vi "File_Write_v2.vi"(0 "Thermocouple Data":dynamicdata(waveform), 1 "Pressure Data":T7, 2 "Use Older File Write?":bool, 3 "Flow Rate Data":cluster{dbl, dbl, dbl, dbl, dbl}, 4 "Raman Data Array":cluster{i32[], i32[]}[](array[cluster]), 5 "Loop Iteration Boolean":bool, 6 "Slave Data Cluster":T5={"Current DoE"=[], "SSI 1 Flow Rate"=0.0, "SSI 2 Flow Rate"=0.0, "FLOM 1 Flow Rate"=0.0, "FLOM 2 Flow Rate"=0.0, "Pumps Running?"=FALSE, "Boolean 2"=FALSE, "Boolean 3"=FALSE, "Boolean 4"=FALSE, "At Equilibrium?"=FALSE, "Script Running?"=FALSE, "Current Script Iteration"=0.0, "Total Script Iterations"=0.0, "FLOM Pumps VISA"="COM2", "SSI 1 Pump VISA"="COM76", "SSI 2 Pump VISA"="COM74", "Huber Unistat VISA"="COM1", "SSI 3 Pump VISA"="COM76", "SSI 4 Pump VISA"="COM76", "SSI 4 Flow Rate"=0.0, "SSI 3 Flow Rate"=0.0, "Flow Meter 1 Rate "=0.0, "Flow Meter 2 Rate"=0.0, "Flow Meter 3 Rate"=0.0, "Flow Meter 4 Rate"=0.0, "SSI 1 Flow Setpoint"=0.0, "SSI 2 Flow Setpoint"=0.0, "SSI 3 Flow Setpoint"=0.0, "SSI 4 Flow Setpoint"=0.0, "Temperature Setpoint"=0.0, "Flow meter 3 COM"=17, "Flow meter 5 COM"=18, "Flow meter 4 COM"=19, "Flow meter 2 COM"=16, "Flow meter 1 COM"=15, "Unit"=enum."PSI", "Pressure COM"="COM6", "Julabo Setpoint"=0.0, "Julabo Control"=enum."Internal", "Overtemp"=50.0, "Subtemp"=-20.0, "HeatMax"=50, "CoolMax"=-100, "InternMax"=50.0, "InternMin"=0.0, "Upper Bandlimit"=100.0, "Lower Bandlimit"=0.0, "Julabo CF41 VISA"="COM3", "Xp (0.6K) Int"=0.6, "Tn (3s) Int"=3, "Tv (0s) Int"=0, "Dynamic (0: aperiodic) Int"=enum."aperiodic", "Xp (0.6K) Ext"=0.6, "Tn (3s) Ext"=3, "Tv (0s) Ext"=0, "XpU (0.6K) Ext"=0.6, "Julabo Serial Configuration"={"Baud Rate"=4800, "Parity"=2, "Data Bits"=7, "Stop Bits"=10, "Flow Control"=2}} {"Julabo Serial Configuration"."Flow Control" items=["None", "XON/XOFF", "RTS/CTS", "XON/XOFF & RTS/CTS", "DTR/DSR", "XON/XOFF & DTR/DSR"]; "Julabo Serial Configuration"."Stop Bits" items=["1.0"=10, "1.5"=15, "2.0"=20]; "Julabo Serial Configuration"."Data Bits" items=["7"=7, "8"=8]; "Julabo Serial Configuration"."Parity" items=["None", "Odd", "Even", "Mark", "Space"]; "Julabo Serial Configuration"."Baud Rate" items=["300"=300, "600"=600, "1200"=1200, "2400"=2400, "4800"=4800, "9600"=9600, "19200"=19200]; "XpU (0.6K) Ext" min=0.1 max=99.9; "Tv (0s) Ext" max=999; "Tn (3s) Ext" min=3 max=9999; "Xp (0.6K) Ext" min=0.1 max=99.9; "Tv (0s) Int" max=999; "Tn (3s) Int" min=3 max=9999; "Xp (0.6K) Int" min=0.1 max=99.9; "Lower Bandlimit" min=0.0 max=200.0; "Upper Bandlimit" min=0.0 max=200.0; "InternMin" format="%.2f"; "InternMax" format="%.2f"; "CoolMax" min=-100 max=0; "HeatMax" max=100; "Subtemp" format="%.2f"; "Overtemp" format="%.2f"; "Julabo Setpoint" format="%.2f"; "Current DoE" format="%0.3f"}, 8 "File Path Cluster":T4, 10 "Julabo Outputs":T1, 12 "Numeric":i32, 13 "Array":i32[](array[numeric]), 14 "Thermocouple T-Plots":T3(graph), 16 "dT/dt":cluster{"dx/dt":dbl, "dx/dt":dbl, "dx/dt":dbl}(graph), 18 "dF/dt":T2(graph)) -> (15 "Data_Reactant 1 path":path caption="selected path", 17 "Data_Reactant 2 path":path caption="selected path", 20 "Filepath Cluster Out":T4, 24 "Data_noRaman path":path caption="selected path", 25 "Data_Product path":path caption="selected path", 27 "Data_Reactant 3 path":path caption="selected path")   [LabVIEW 2015]
uses:
  --Controls and TypeDefs--/DoE_Control_Cluster.ctl
  <instrlib>/JULABO DeviceDriver/Examples/Julabo Serial Control.ctl
  <vilib>/Utility/file.llb/Write To Spreadsheet File (string).vi
panel:
  in  "Write Raman-Appended Files?":bool
  in  "data File Header":string[][](table)=[["Time"], ["TC1"], ["TC2"], ["TC3"], ["TC1 SG Filter"], ["TC2 SG Filter"], ["TC3 SG Filter"], ["TC1 dT/dt"], ["TC2 dT/dt"], ["TC3 dT/dt"], ["P1"], ["P2"], ["P3"], ["P4"], ["Fset1"], ["Fset2"], ["Fset3"], ["Fset4"], ["F1"], ["F2"], ["F3"], ["F4"], ["F5"], ["F1 dF/dt"], ["F2 dF/dt"], ["F3 dF/dt"], ["F4 dF/dt"], ["F5 dF/dt"]]
  # "Julabo"
  # "Limits"
  # "PID Control Parameters"
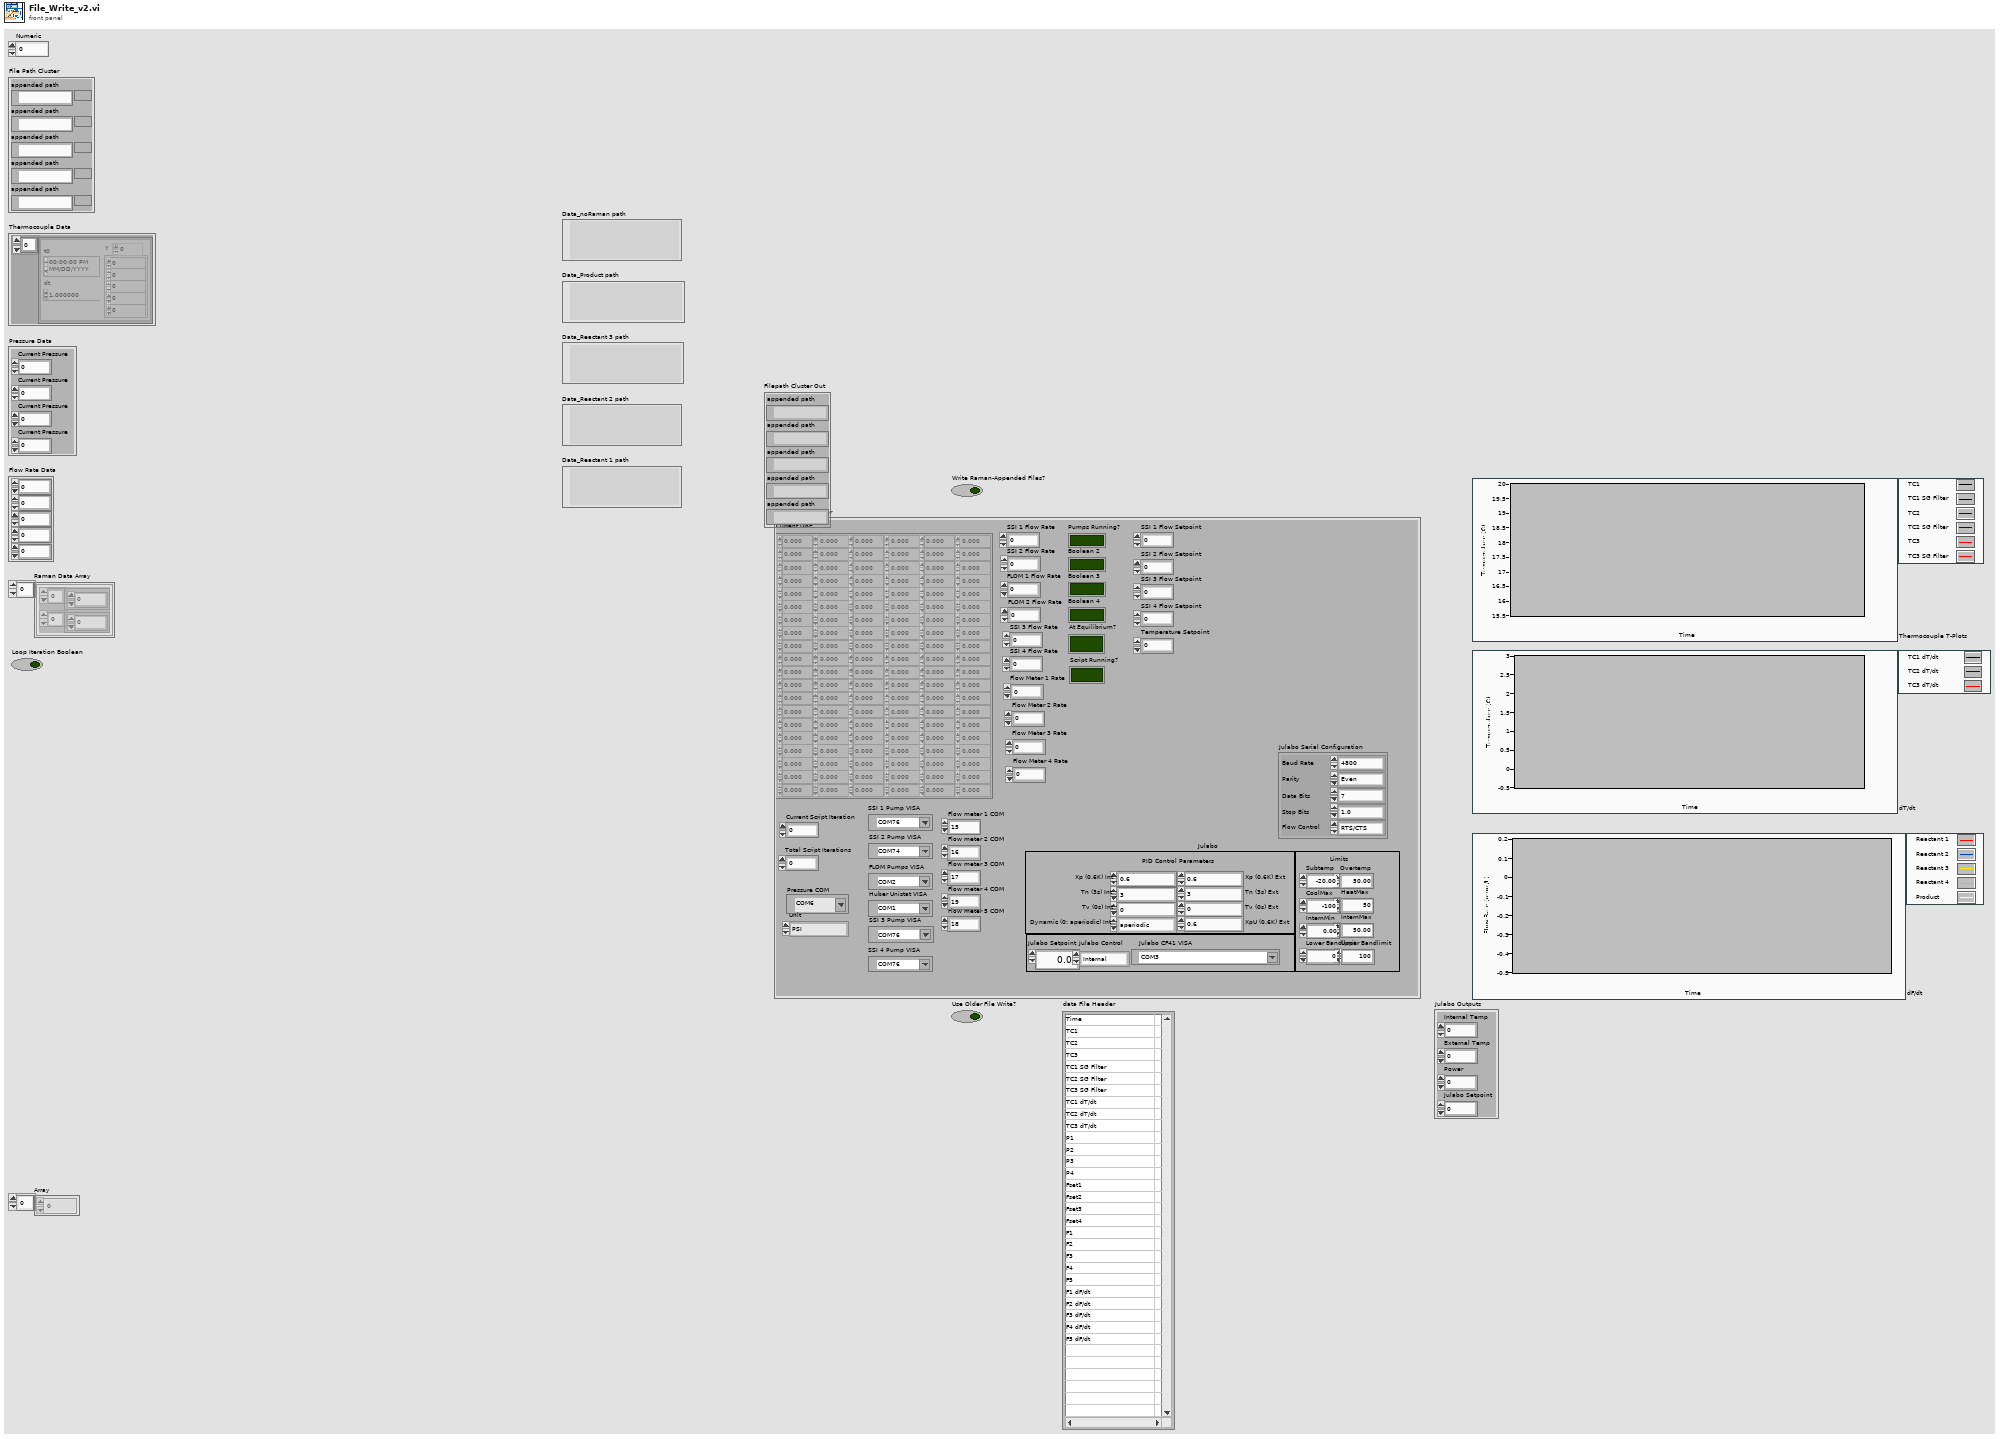
[diagram p1: front panel]
types:
  T1 = cluster{"Internal Temp":dbl, "External Temp":dbl, "Power":i8, "Julabo Setpoint":dbl}
  T2 = cluster{"MeasureResult Scaled":dbl, "MeasureResult Scaled":dbl, "MeasureResult Scaled":dbl, "MeasureResult Scaled":dbl, "MeasureResult Scaled":dbl}
  T3 = cluster{dbl, "Filtered x":dbl, dbl, "Filtered x":dbl, dbl, "Filtered x":dbl}
  T4 = cluster{"appended path":path, "appended path":path, "appended path":path, "appended path":path, "appended path":path}
  T5 = typedef "DoE_Control_Cluster.ctl" = cluster{"Current DoE":dbl[][], "SSI 1 Flow Rate":dbl, "SSI 2 Flow Rate":dbl, "FLOM 1 Flow Rate":dbl, "FLOM 2 Flow Rate":dbl, "Pumps Running?":bool, "Boolean 2":bool, "Boolean 3":bool, "Boolean 4":bool, "At Equilibrium?":bool, "Script Running?":bool, "Current Script Iteration":dbl, "Total Script Iterations":dbl, "FLOM Pumps VISA":refnum<visa-resource-name>, "SSI 1 Pump VISA":refnum<visa-resource-name>, "SSI 2 Pump VISA":refnum<visa-resource-name>, "Huber Unistat VISA":refnum<visa-resource-name>, "SSI 3 Pump VISA":refnum<visa-resource-name>, "SSI 4 Pump VISA":refnum<visa-resource-name>, "SSI 4 Flow Rate":dbl, "SSI 3 Flow Rate":dbl, "Flow Meter 1 Rate ":dbl, "Flow Meter 2 Rate":dbl, "Flow Meter 3 Rate":dbl, "Flow Meter 4 Rate":dbl, "SSI 1 Flow Setpoint":dbl, "SSI 2 Flow Setpoint":dbl, "SSI 3 Flow Setpoint":dbl, "SSI 4 Flow Setpoint":dbl, "Temperature Setpoint":dbl, "Flow meter 3 COM":u16, "Flow meter 5 COM":u16, "Flow meter 4 COM":u16, "Flow meter 2 COM":u16, "Flow meter 1 COM":u16, "Unit":enum16{"PSI", "Bar", "cm H2O", "ft H2O", "hectoPascal", "in Hg", "in H2O", "kiloPascal", "milliBar", "mmHg", "MegaPascal", "Numeric Pressure"}, "Pressure COM":refnum<visa-resource-name>, "Julabo Setpoint":dbl, "Julabo Control":enum16{"Internal", "External"}, "Overtemp":dbl, "Subtemp":dbl, "HeatMax":u8, "CoolMax":i8, "InternMax":dbl, "InternMin":dbl, "Upper Bandlimit":dbl, "Lower Bandlimit":dbl, "Julabo CF41 VISA":refnum<visa-resource-name>, "Xp (0.6K) Int":dbl, "Tn (3s) Int":u16, "Tv (0s) Int":u16, "Dynamic (0: aperiodic) Int":enum16{"aperiodic", "standard"}, "Xp (0.6K) Ext":dbl, "Tn (3s) Ext":u16, "Tv (0s) Ext":u16, "XpU (0.6K) Ext":dbl, "Julabo Serial Configuration":T6}
  T6 = typedef "Julabo Serial Control.ctl" = cluster{"Baud Rate":u32, "Parity":u16, "Data Bits":u16, "Stop Bits":u16, "Flow Control":u16}
  T7 = cluster{"Current Pressure":dbl, "Current Pressure":dbl, "Current Pressure":dbl, "Current Pressure":dbl}
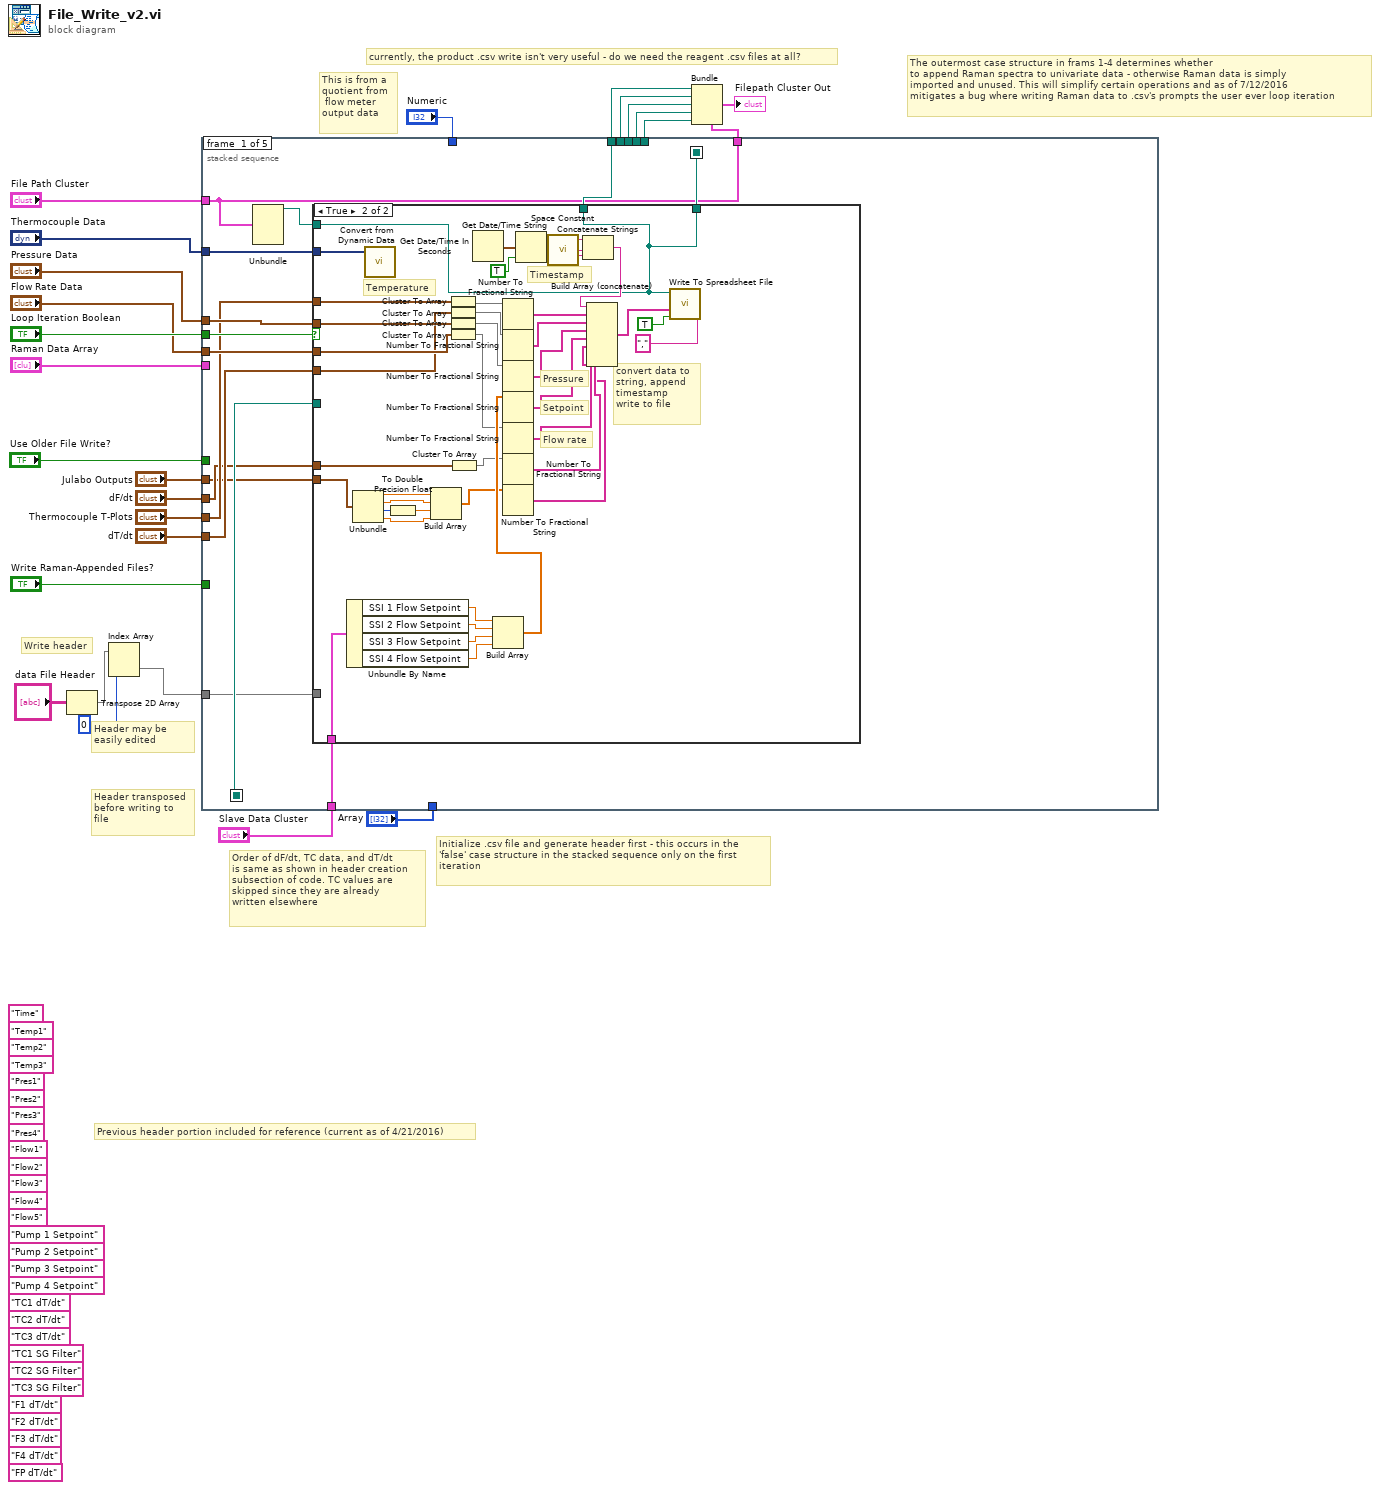
[diagram p0: block diagram]
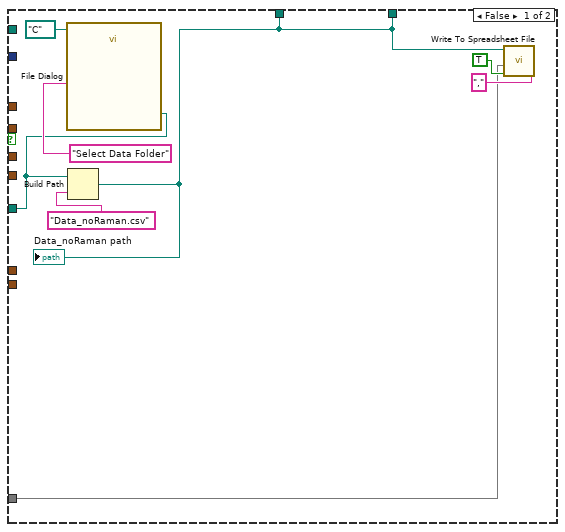
[diagram p2: hidden frame]
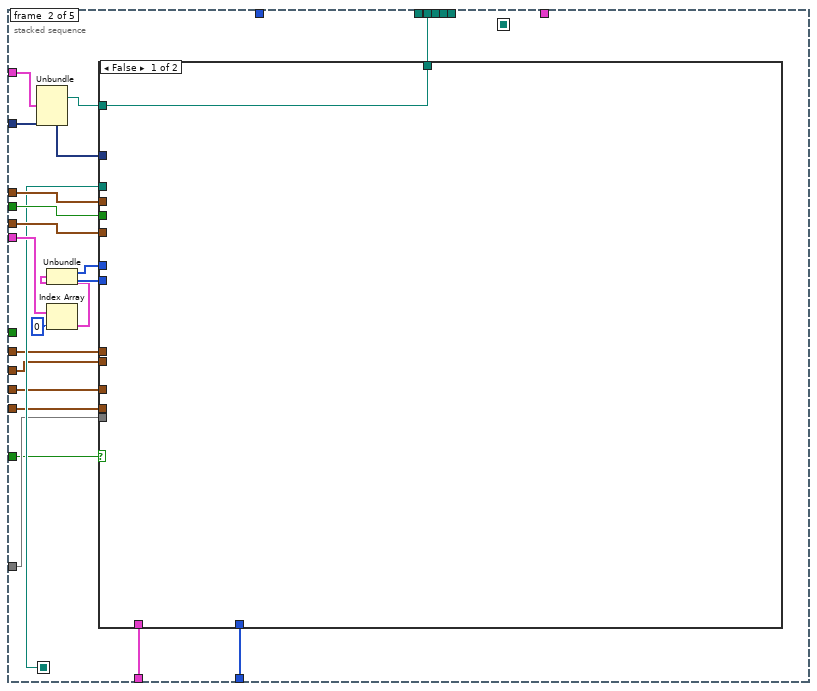
[diagram p3: hidden frame]
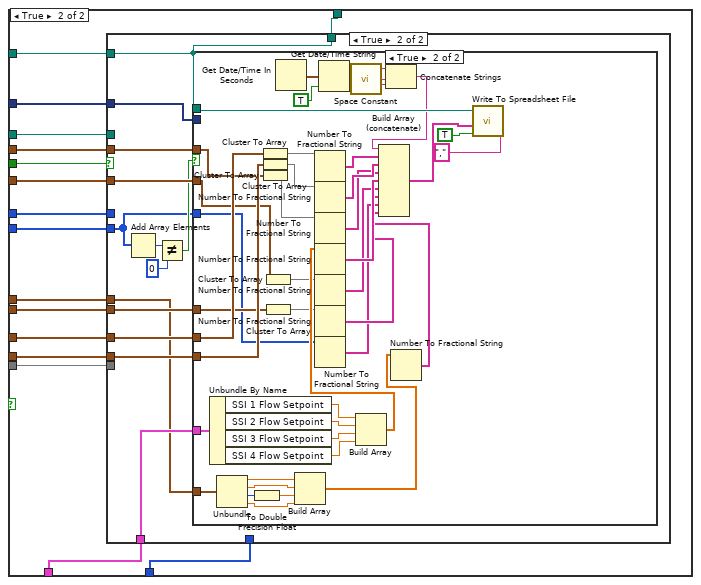
[diagram p4: hidden frame]
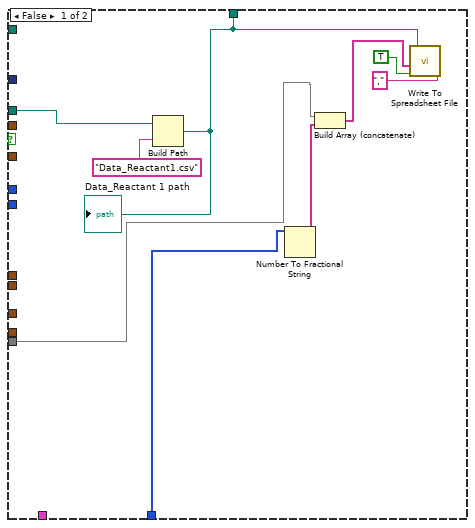
[diagram p5: hidden frame]
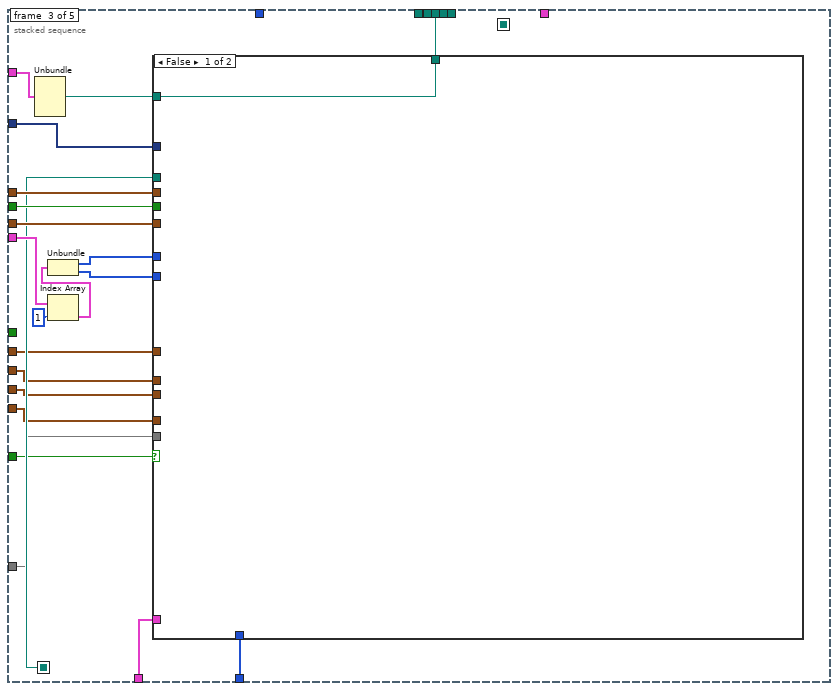
[diagram p7: hidden frame]
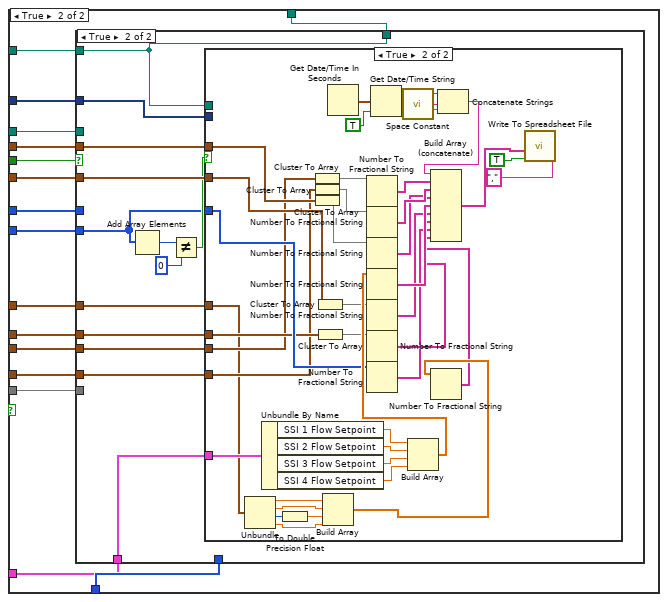
[diagram p8: hidden frame]
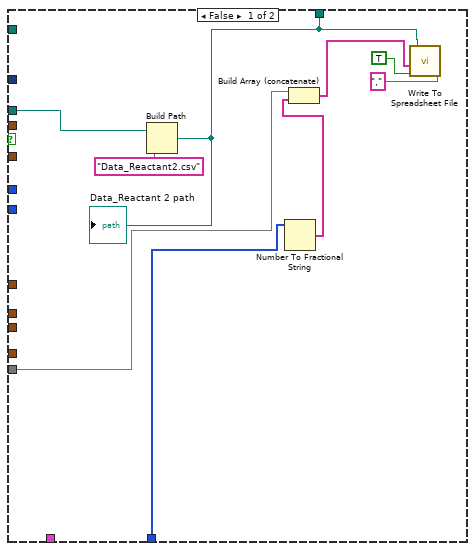
[diagram p9: hidden frame]
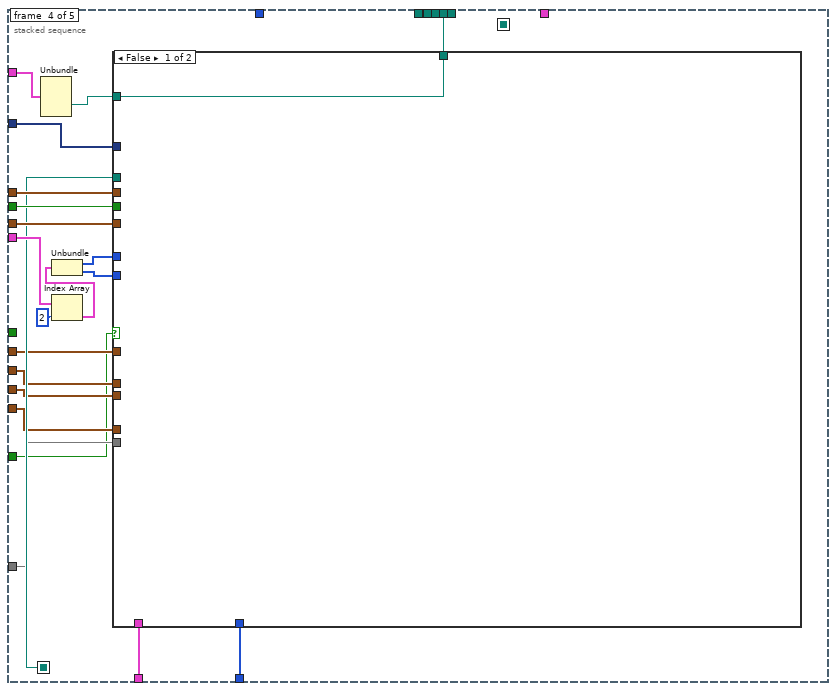
[diagram p11: hidden frame]
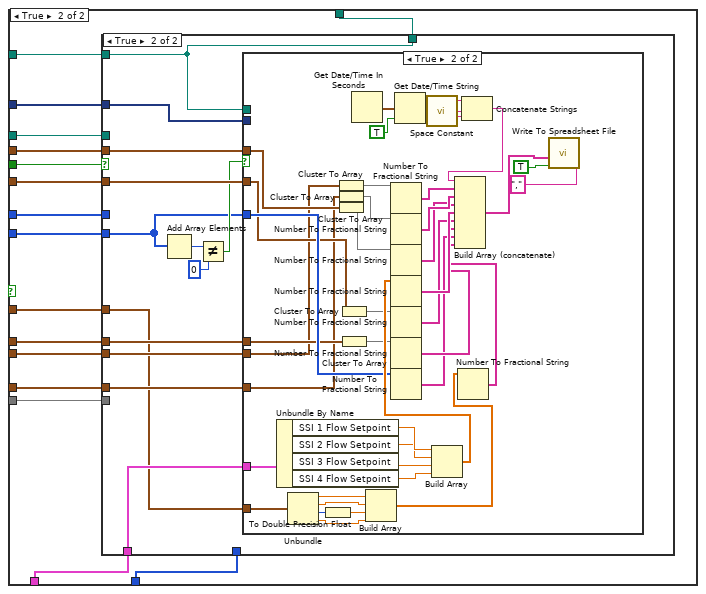
[diagram p12: hidden frame]
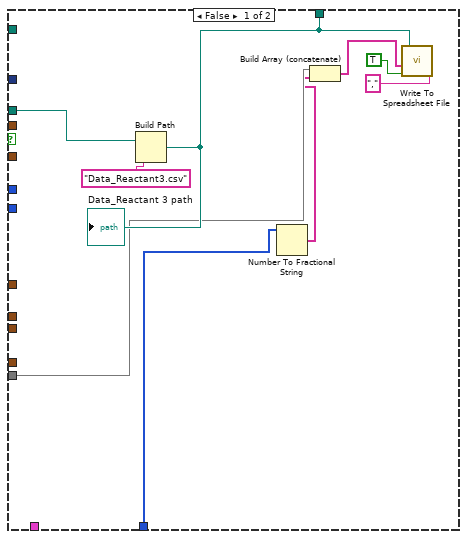
[diagram p13: hidden frame]
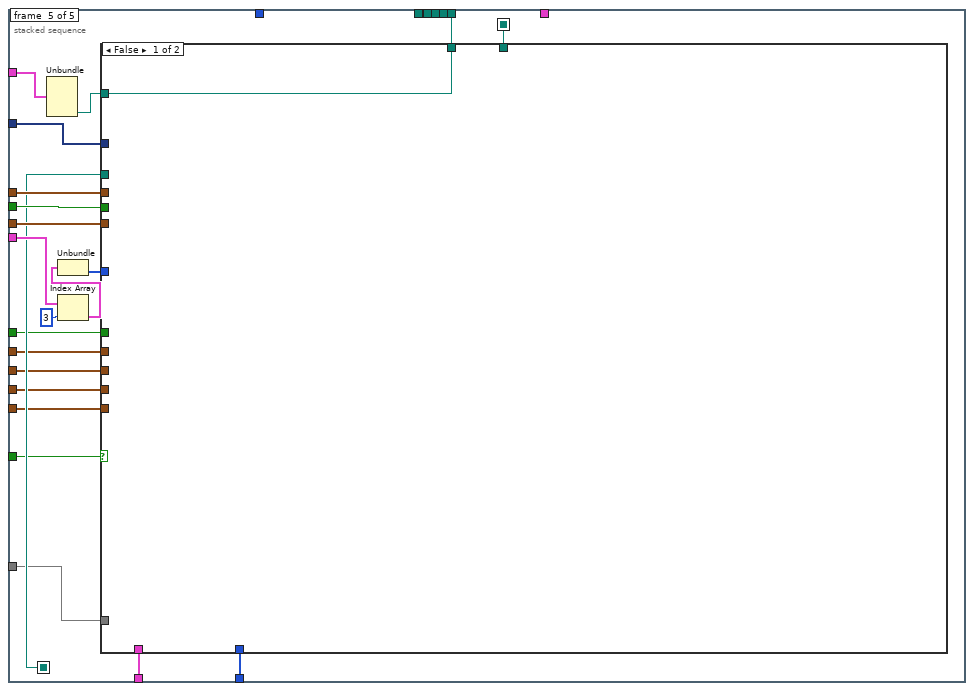
[diagram p15: hidden frame]
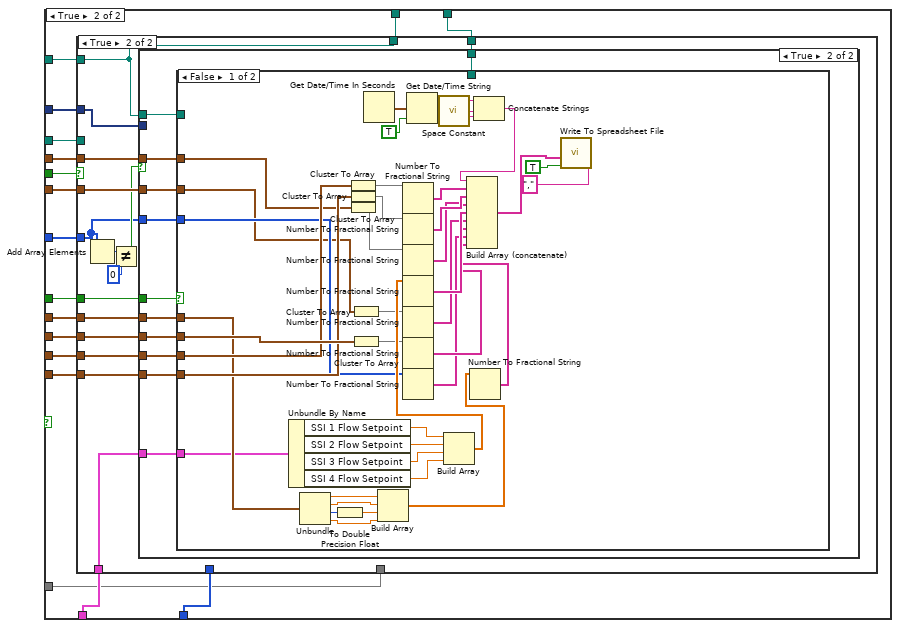
[diagram p16: hidden frame]
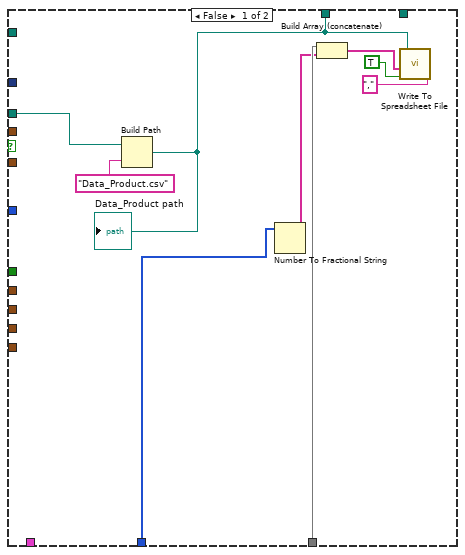
[diagram p17: hidden frame]
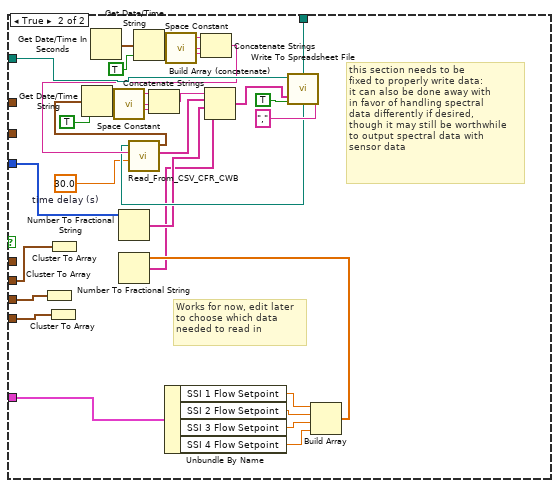
[diagram p19: hidden frame]
diagram:
  (unwired) "FP dT/dt"
  (unwired) "F4 dT/dt"
  (unwired) "F3 dT/dt"
  (unwired) "F2 dT/dt"
  (unwired) "F1 dT/dt"
  (unwired) "TC2 SG Filter"
  (unwired) "TC3 SG Filter"
  (unwired) "TC1 SG Filter"
  (unwired) "TC3 dT/dt"
  (unwired) "TC2 dT/dt"
  (unwired) "TC1 dT/dt"
  (unwired) "Pump 4 Setpoint"
  (unwired) "Pump 3 Setpoint"
  (unwired) "Pump 2 Setpoint"
  (unwired) "Pump 1 Setpoint"
  (unwired) "Flow5" ("delimiter (\\t)")
  (unwired) "Flow4" ("delimiter (\\t)")
  (unwired) "Flow3" ("delimiter (\\t)")
  (unwired) "Flow2" ("delimiter (\\t)")
  (unwired) "Flow1" ("delimiter (\\t)")
  (unwired) "Pres4" ("delimiter (\\t)")
  (unwired) "Pres3" ("delimiter (\\t)")
  (unwired) "Pres2" ("delimiter (\\t)")
  (unwired) "Pres1" ("delimiter (\\t)")
  (unwired) "Temp3" ("delimiter (\\t)")
  (unwired) "Temp2" ("delimiter (\\t)")
  (unwired) "Temp1" ("delimiter (\\t)")
  (unwired) "Time" ("delimiter (\\t)")
  # "The outermost case structure in frams 1-4 determines whether\nto append Raman spectra to univariate data - otherwise Raman data is simply\nimported and unused. This will simplify certain operations and as of 7/12/2016 \nmitigates a bug where writing Raman data to .csv's prompts the user ever loop iteration"
  # "currently, the product .csv write isn't very useful - do we need the reagent .csv files at all?"
  # "Write header"
  # "Previous header portion included for reference (current as of 4/21/2016)"
  # "Header transposed\nbefore writing to \nfile"
  # "Header may be \neasily edited"
  # "Order of dF/dt, TC data, and dT/dt \nis same as shown in header creation \nsubsection of code. TC values are\nskipped since they are already\nwritten elsewhere"
  # "Initialize .csv file and generate header first - this occurs in the 'false' case structure in the stacked sequence only on the first iteration"
  # "This is from a \nquotient from\n flow meter\noutput data"
  n1 = Transpose 2D Array(2D array="data File Header") -> (transposed array=w6:string[][])
  n2 = Index Array(array=w6, index (row)=0) -> (element=w5:string[])  [unwired: 1 in]
  n3 = stacked-sequence {
    seq-local: [w36 _ _ _ _] -> [_ w99 w201 w302 w405]
    seq-local: [w35 _ _ _ _] -> [_ _ _ _ w403]
    tunnel: "Thermocouple Data" -> [w37 w111 w213 w314 w416]
    tunnel: "Pressure Data" -> [w41 w110 w212 w313 w415]
    tunnel: "Flow Rate Data" -> [w40 w109 w211 w312 w414]
    tunnel: "Loop Iteration Boolean" -> [w39 w108 w210 w311 w413]
    tunnel: [w33 _ _ _ _] -> w15
    tunnel: "File Path Cluster" -> [w32 w101 w203 w304 w407]
    tunnel: "Raman Data Array" -> [_ w105 w207 w308 w411]
    tunnel: [_ w102 _ _ _] -> w14
    tunnel: [_ _ w204 _ _] -> w13
    tunnel: [_ _ _ w305 _] -> w11
    tunnel: [_ _ _ _ w408] -> w12
    tunnel: "Array" -> [_ w98 w200 w301 w404]
    tunnel: "Numeric" -> [_ _ _ _ _]
    tunnel: "Slave Data Cluster" -> [w34 w97 w199 w300 w402]
    tunnel: [w32 _ _ _ _] -> w17
    tunnel: "dT/dt" -> [w29 w94 w196 w297 w401]
    tunnel: "Thermocouple T-Plots" -> [w30 w95 w195 w296 w400]
    tunnel: "dF/dt" -> [w28 w93 w197 w298 w399]
    tunnel: w5 -> [w31 w96 w198 w299 w398]
    tunnel: "Julabo Outputs" -> [w27 w92 w194 w295 w397]
    tunnel: "Use Older File Write?" -> [_ _ _ _ w396]
    tunnel: "Write Raman-Appended Files?" -> [_ w91 w193 w294 w395]
    frame #0 {
      n4 = Unbundle(w32) -> ("appended path"=w38:path)  [unwired: 4 out]
      n5 = case shown="True" w39 {
        tunnel: w37 -> [_ w79]
        tunnel: w41 -> [_ w78]
        tunnel: w40 -> [_ w77]
        tunnel: w38 -> [_ w76]
        tunnel: [w43 w76] -> w33
        tunnel: [w44 _] -> w36
        tunnel: [w43 w76] -> w35
        tunnel: w34 -> [_ w75]
        tunnel: w31 -> [w42 _]
        tunnel: w30 -> [_ w70]
        tunnel: w29 -> [_ w68]
        tunnel: w28 -> [_ w61]
        tunnel: w27 -> [_ w57]
        frame False {
          n6 = call "File Dialog"("start path"=path "C:/", "prompt"="Select Data Folder") -> ("selected path"=w44:path)  [unwired: 10 in, 3 out]
          n7 = Build Path(base path=w44, name or relative path="Data_noRaman.csv" ("default name")) -> (appended path=w43:path)
          "Data_noRaman path" <- w43
          n8 = call-poly <vilib>:"Write To Spreadsheet File.vi"("delimiter (\\t)"="," ("delimiter (\\t)"), "append to file? (new file:F)"=TRUE ("append to file?"), "1D data"=w42, "file path (dialog if empty)"=w43) -> ()  [unwired: 4 in, 1 out]
        }
        frame True {
          # "Timestamp"
          # "Setpoint"
          # "Temperature"
          # "Pressure"
          # "Flow rate"
          # "convert data to \nstring, append\ntimestamp\nwrite to file"
          n9 = Unbundle By Name(w75) -> ("SSI 1 Flow Setpoint"=w74:dbl, "SSI 2 Flow Setpoint"=w73:dbl, "SSI 3 Flow Setpoint"=w72:dbl, "SSI 4 Flow Setpoint"=w71:dbl)
          n10 = Unbundle(w57) -> ("Internal Temp"=w55:dbl, "External Temp"=w54:dbl, "Power"=w56:i8, "Julabo Setpoint"=w52:dbl)
          n11 = call "Convert from Dynamic Data"("Dynamic Data Type"=w79) -> ()  [unwired: 3 in, 1 out]
          n12 = To Double Precision Float(number=w56) -> (double precision float=w53:dbl)
          n13 = Build Array(w55, w54, w53, w52) -> (w51:dbl[])
          n14 = Cluster To Array(cluster=w70) -> (array=w69:dbl[])
          n15 = Cluster To Array(cluster=w68) -> (array=w67:dbl[])
          n16 = Cluster To Array(cluster=w78) -> (array=w88:dbl[])
          n17 = Cluster To Array(cluster=w77) -> (array=w64:dbl[])
          n18 = Cluster To Array(cluster=w61) -> (array=w60:dbl[])
          n19 = Get Date/Time In Seconds() -> (seconds since 1Jan1904=w82:timestamp)
          n20 = Build Array(w74, w73, w72, w71) -> (w65:dbl[])
          n21 = Number To Fractional String(number=w69) -> (F-format string=w89:string[])  [unwired: 3 in]
          n22 = Number To Fractional String(number=w67) -> (F-format string=w66:string[])  [unwired: 3 in]
          n23 = Number To Fractional String(number=w88) -> (F-format string=w63:string[])  [unwired: 3 in]
          n24 = Number To Fractional String(number=w65) -> (F-format string=w62:string[])  [unwired: 3 in]
          n25 = Number To Fractional String(number=w64) -> (F-format string=w59:string[])  [unwired: 3 in]
          n26 = Number To Fractional String(number=w60) -> (F-format string=w58:string[])  [unwired: 3 in]
          n27 = Number To Fractional String(number=w51) -> (F-format string=w50:string[])  [unwired: 3 in]
          n28 = Get Date/Time String(seconds (now)=w82, want seconds? (F)=TRUE) -> (date string=w84:string, time string=w85:string)  [unwired: 1 in]
          n29 = call <vilib>:"Space Constant.vi"() -> ("String"=w86:string)
          n30 = Concatenate Strings(w84, w86, w85) -> (w87:string)
          n31 = Build Array (concatenate)(w87, w89, w66, w63, w62, w59, w58, w50) -> (w90:string[])
          n32 = call-poly <vilib>:"Write To Spreadsheet File.vi"("delimiter (\\t)"="," ("delimiter (\\t)"), "append to file? (new file:F)"=TRUE ("append to file?"), "1D data"=w90, "file path (dialog if empty)"=w76) -> ()  [unwired: 4 in, 1 out]
        }
      }
    }
    frame #1 {
      n33 = Unbundle(w101) -> ("appended path"=w100:path)  [unwired: 4 out]
      n34 = Index Array(array=w105, index=0) -> (element=w104:cluster{i32[], i32[]})
      n35 = Unbundle(w104) -> (w106:i32[], w107:i32[])
      n36 = case shown="False" w91 {
        tunnel: w111 -> [_ w128]
        tunnel: w110 -> [_ w127]
        tunnel: w109 -> [_ w126]
        tunnel: w108 -> [_ w125]
        tunnel: w107 -> [_ w124]
        tunnel: w106 -> [_ w123]
        tunnel: [w112 w122] -> w102
        tunnel: w100 -> [w112 w121]
        tunnel: w99 -> [_ w120]
        tunnel: w98 -> [_ w119]
        tunnel: w97 -> [_ w118]
        tunnel: w96 -> [_ w117]
        tunnel: w95 -> [_ w116]
        tunnel: w94 -> [_ w115]
        tunnel: w93 -> [_ w114]
        tunnel: w92 -> [_ w113]
        frame False {
        }
        frame True {
          n37 = case shown="True" w125 {
            tunnel: w128 -> [_ w150]
            tunnel: w127 -> [_ w149]
            tunnel: w126 -> [_ w148]
            tunnel: w121 -> [_ w147]
            tunnel: [w137 w147] -> w122
            tunnel: w124 -> [_ w143]
            tunnel: w123 -> [_ _]
            tunnel: w120 -> [w136 _]
            tunnel: w119 -> [w132 _]
            tunnel: w118 -> [_ w142]
            tunnel: w117 -> [w131 _]
            tunnel: w116 -> [_ w141]
            tunnel: w115 -> [_ w140]
            tunnel: w114 -> [_ w139]
            tunnel: w113 -> [_ w138]
            frame False {
              n38 = Build Path(base path=w136, name or relative path="Data_Reactant1.csv" ("default name")) -> (appended path=w137:path)
              "Data_Reactant 1 path" <- w137
              n39 = Number To Fractional String(number=w132) -> (F-format string=w130:string[])  [unwired: 3 in]
              n40 = Build Array (concatenate)(w131, w130) -> (w129:string[])
              n41 = call-poly <vilib>:"Write To Spreadsheet File.vi"("delimiter (\\t)"="," ("delimiter (\\t)"), "append to file? (new file:F)"=TRUE ("append to file?"), "1D data"=w129, "file path (dialog if empty)"=w137) -> ()  [unwired: 4 in, 1 out]
            }
            frame True {
              n42 = Add Array Elements(numeric array=w143) -> (sum=w146:i32)
              n43 = Not Equal?(x=w146, y=0) -> (x != y?=w144:bool)
              n44 = case shown="True" w144 {
                tunnel: w150 -> [_ _]
                tunnel: w149 -> [_ w173]
                tunnel: w148 -> [_ w168]
                tunnel: w147 -> [_ w185]
                tunnel: w143 -> [_ w162]
                tunnel: w142 -> [_ w160]
                tunnel: w141 -> [_ w179]
                tunnel: w140 -> [_ w176]
                tunnel: w139 -> [_ w165]
                tunnel: w138 -> [_ w153]
                frame False {
                }
                frame True {
                  n45 = Unbundle By Name(w160) -> ("SSI 1 Flow Setpoint"=w184:dbl, "SSI 2 Flow Setpoint"=w183:dbl, "SSI 3 Flow Setpoint"=w182:dbl, "SSI 4 Flow Setpoint"=w181:dbl)
                  n46 = Unbundle(w153) -> ("Internal Temp"=w157:dbl, "External Temp"=w156:dbl, "Power"=w158:i8, "Julabo Setpoint"=w154:dbl)
                  n47 = To Double Precision Float(number=w158) -> (double precision float=w155:dbl)
                  n48 = Cluster To Array(cluster=w179) -> (array=w178:dbl[])
                  n49 = Cluster To Array(cluster=w176) -> (array=w175:dbl[])
                  n50 = Cluster To Array(cluster=w173) -> (array=w172:dbl[])
                  n51 = Cluster To Array(cluster=w168) -> (array=w167:dbl[])
                  n52 = Cluster To Array(cluster=w165) -> (array=w164:dbl[])
                  n53 = Get Date/Time In Seconds() -> (seconds since 1Jan1904=w188:timestamp)
                  n54 = Build Array(w157, w156, w155, w154) -> (w152:dbl[])
                  n55 = Number To Fractional String(number=w178) -> (F-format string=w177:string[])  [unwired: 3 in]
                  n56 = Number To Fractional String(number=w175) -> (F-format string=w174:string[])  [unwired: 3 in]
                  n57 = Number To Fractional String(number=w172) -> (F-format string=w171:string[])  [unwired: 3 in]
                  n58 = Number To Fractional String(number=w167) -> (F-format string=w166:string[])  [unwired: 3 in]
                  n59 = Number To Fractional String(number=w164) -> (F-format string=w163:string[])  [unwired: 3 in]
                  n60 = Number To Fractional String(number=w162) -> (F-format string=w161:string[])  [unwired: 3 in]
                  n61 = Get Date/Time String(seconds (now)=w188, want seconds? (F)=TRUE) -> (date string=w190:string, time string=w191:string)  [unwired: 1 in]
                  n62 = call <vilib>:"Space Constant.vi"() -> ("String"=w192:string)
                  n63 = Build Array(w184, w183, w182, w181) -> (w170:dbl[])
                  n64 = Number To Fractional String(number=w170) -> (F-format string=w169:string[])  [unwired: 3 in]
                  n65 = Concatenate Strings(w190, w192, w191) -> (w180:string)
                  n66 = Number To Fractional String(number=w152) -> (F-format string=w151:string[])  [unwired: 3 in]
                  n67 = Build Array (concatenate)(w180, w177, w174, w171, w169, w166, w163, w161, w151) -> (w159:string[])
                  n68 = call-poly <vilib>:"Write To Spreadsheet File.vi"("delimiter (\\t)"="," ("delimiter (\\t)"), "append to file? (new file:F)"=TRUE ("append to file?"), "1D data"=w159, "file path (dialog if empty)"=w185) -> ()  [unwired: 4 in, 1 out]
                }
              }
            }
          }
        }
      }
    }
    frame #2 {
      n69 = Unbundle(w203) -> ("appended path"=w202:path)  [unwired: 4 out]
      n70 = Index Array(array=w207, index=1) -> (element=w206:cluster{i32[], i32[]})
      n71 = Unbundle(w206) -> (w208:i32[], w209:i32[])
      n72 = case shown="False" w193 {
        tunnel: w213 -> [_ w230]
        tunnel: w212 -> [_ w229]
        tunnel: w211 -> [_ w228]
        tunnel: w210 -> [_ w227]
        tunnel: w209 -> [_ w226]
        tunnel: w208 -> [_ w225]
        tunnel: [w214 w224] -> w204
        tunnel: w202 -> [w214 w223]
        tunnel: w201 -> [_ w222]
        tunnel: w200 -> [_ w221]
        tunnel: w199 -> [_ w220]
        tunnel: w198 -> [_ w219]
        tunnel: w197 -> [_ w218]
        tunnel: w196 -> [_ w217]
        tunnel: w195 -> [_ w216]
        tunnel: w194 -> [_ w215]
        frame False {
        }
        frame True {
          n73 = case shown="True" w227 {
            tunnel: w230 -> [_ w252]
            tunnel: w229 -> [_ w251]
            tunnel: w228 -> [_ w250]
            tunnel: w223 -> [_ w249]
            tunnel: [w239 w249] -> w224
            tunnel: w226 -> [_ w245]
            tunnel: w225 -> [_ _]
            tunnel: w222 -> [w238 _]
            tunnel: w221 -> [w234 _]
            tunnel: w220 -> [_ w244]
            tunnel: w219 -> [w233 _]
            tunnel: w218 -> [_ w243]
            tunnel: w217 -> [_ w242]
            tunnel: w216 -> [_ w241]
            tunnel: w215 -> [_ w240]
            frame False {
              n74 = Build Path(base path=w238, name or relative path="Data_Reactant2.csv" ("default name")) -> (appended path=w239:path)
              "Data_Reactant 2 path" <- w239
              n75 = Number To Fractional String(number=w234) -> (F-format string=w232:string[])  [unwired: 3 in]
              n76 = Build Array (concatenate)(w233, w232) -> (w231:string[])
              n77 = call-poly <vilib>:"Write To Spreadsheet File.vi"("delimiter (\\t)"="," ("delimiter (\\t)"), "append to file? (new file:F)"=TRUE ("append to file?"), "1D data"=w231, "file path (dialog if empty)"=w239) -> ()  [unwired: 4 in, 1 out]
            }
            frame True {
              n78 = Add Array Elements(numeric array=w245) -> (sum=w248:i32)
              n79 = Not Equal?(x=w248, y=0) -> (x != y?=w246:bool)
              n80 = case shown="True" w246 {
                tunnel: w252 -> [_ _]
                tunnel: w251 -> [_ w264]
                tunnel: w250 -> [_ w265]
                tunnel: w249 -> [_ _]
                tunnel: w245 -> [_ w267]
                tunnel: w244 -> [_ w268]
                tunnel: w243 -> [_ w266]
                tunnel: w242 -> [_ w263]
                tunnel: w241 -> [_ w262]
                tunnel: w240 -> [_ w255]
                frame False {
                }
                frame True {
                  n81 = Unbundle(w255) -> ("Internal Temp"=w259:dbl, "External Temp"=w258:dbl, "Power"=w260:i8, "Julabo Setpoint"=w256:dbl)
                  n82 = Unbundle By Name(w268) -> ("SSI 1 Flow Setpoint"=w286:dbl, "SSI 2 Flow Setpoint"=w285:dbl, "SSI 3 Flow Setpoint"=w284:dbl, "SSI 4 Flow Setpoint"=w283:dbl)
                  n83 = To Double Precision Float(number=w260) -> (double precision float=w257:dbl)
                  n84 = Cluster To Array(cluster=w262) -> (array=w281:dbl[])
                  n85 = Cluster To Array(cluster=w263) -> (array=w279:dbl[])
                  n86 = Cluster To Array(cluster=w264) -> (array=w277:dbl[])
                  n87 = Cluster To Array(cluster=w265) -> (array=w273:dbl[])
                  n88 = Cluster To Array(cluster=w266) -> (array=w271:dbl[])
                  n89 = Build Array(w259, w258, w257, w256) -> (w254:dbl[])
                  n90 = Get Date/Time In Seconds() -> (seconds since 1Jan1904=w289:timestamp)
                  n91 = Number To Fractional String(number=w281) -> (F-format string=w280:string[])  [unwired: 3 in]
                  n92 = Number To Fractional String(number=w279) -> (F-format string=w278:string[])  [unwired: 3 in]
                  n93 = Number To Fractional String(number=w277) -> (F-format string=w276:string[])  [unwired: 3 in]
                  n94 = Number To Fractional String(number=w273) -> (F-format string=w272:string[])  [unwired: 3 in]
                  n95 = Number To Fractional String(number=w271) -> (F-format string=w270:string[])  [unwired: 3 in]
                  n96 = Number To Fractional String(number=w267) -> (F-format string=w269:string[])  [unwired: 3 in]
                  n97 = Get Date/Time String(seconds (now)=w289, want seconds? (F)=TRUE) -> (date string=w291:string, time string=w292:string)  [unwired: 1 in]
                  n98 = call <vilib>:"Space Constant.vi"() -> ("String"=w293:string)
                  n99 = Build Array(w286, w285, w284, w283) -> (w275:dbl[])
                  n100 = Number To Fractional String(number=w275) -> (F-format string=w274:string[])  [unwired: 3 in]
                  n101 = Number To Fractional String(number=w254) -> (F-format string=w253:string[])  [unwired: 3 in]
                  n102 = Concatenate Strings(w291, w293, w292) -> (w282:string)
                  n103 = Build Array (concatenate)(w282, w280, w278, w276, w274, w272, w270, w269, w253) -> (w261:string[])
                  n104 = call-poly <vilib>:"Write To Spreadsheet File.vi"("delimiter (\\t)"="," ("delimiter (\\t)"), "append to file? (new file:F)"=TRUE ("append to file?"), "1D data"=w261) -> ()  [unwired: 5 in, 1 out]
                }
              }
            }
          }
        }
      }
    }
    frame #3 {
      n105 = Unbundle(w304) -> ("appended path"=w303:path)  [unwired: 4 out]
      n106 = Index Array(array=w308, index=2) -> (element=w307:cluster{i32[], i32[]})
      n107 = Unbundle(w307) -> (w309:i32[], w310:i32[])
      n108 = case shown="False" w294 {
        tunnel: w314 -> [_ w331]
        tunnel: w313 -> [_ w330]
        tunnel: w312 -> [_ w329]
        tunnel: w311 -> [_ w328]
        tunnel: w310 -> [_ w327]
        tunnel: w309 -> [_ w326]
        tunnel: [w315 w325] -> w305
        tunnel: w303 -> [w315 w324]
        tunnel: w302 -> [_ w323]
        tunnel: w301 -> [_ w322]
        tunnel: w300 -> [_ w321]
        tunnel: w299 -> [_ w320]
        tunnel: w298 -> [_ w319]
        tunnel: w297 -> [_ w318]
        tunnel: w296 -> [_ w317]
        tunnel: w295 -> [_ w316]
        frame False {
        }
        frame True {
          n109 = case shown="True" w328 {
            tunnel: w331 -> [_ w353]
            tunnel: w330 -> [_ w352]
            tunnel: w329 -> [_ w351]
            tunnel: w324 -> [_ w350]
            tunnel: [w340 w350] -> w325
            tunnel: w327 -> [_ w346]
            tunnel: w326 -> [_ _]
            tunnel: w323 -> [w339 _]
            tunnel: w322 -> [w335 _]
            tunnel: w321 -> [_ w345]
            tunnel: w320 -> [w334 _]
            tunnel: w319 -> [_ w344]
            tunnel: w318 -> [_ w343]
            tunnel: w317 -> [_ w342]
            tunnel: w316 -> [_ w341]
            frame False {
              n110 = Build Path(base path=w339, name or relative path="Data_Reactant3.csv" ("default name")) -> (appended path=w340:path)
              "Data_Reactant 3 path" <- w340
              n111 = Number To Fractional String(number=w335) -> (F-format string=w333:string[])  [unwired: 3 in]
              n112 = Build Array (concatenate)(w334, w333) -> (w332:string[])
              n113 = call-poly <vilib>:"Write To Spreadsheet File.vi"("delimiter (\\t)"="," ("delimiter (\\t)"), "append to file? (new file:F)"=TRUE ("append to file?"), "1D data"=w332, "file path (dialog if empty)"=w340) -> ()  [unwired: 4 in, 1 out]
            }
            frame True {
              n114 = Add Array Elements(numeric array=w346) -> (sum=w349:i32)
              n115 = Not Equal?(x=w349, y=0) -> (x != y?=w347:bool)
              n116 = case shown="True" w347 {
                tunnel: w353 -> [_ _]
                tunnel: w352 -> [_ w364]
                tunnel: w351 -> [_ w365]
                tunnel: w350 -> [_ _]
                tunnel: w346 -> [_ w367]
                tunnel: w345 -> [_ w368]
                tunnel: w344 -> [_ w366]
                tunnel: w343 -> [_ w363]
                tunnel: w342 -> [_ w362]
                tunnel: w341 -> [_ w356]
                frame False {
                }
                frame True {
                  n117 = Unbundle By Name(w368) -> ("SSI 1 Flow Setpoint"=w387:dbl, "SSI 2 Flow Setpoint"=w386:dbl, "SSI 3 Flow Setpoint"=w385:dbl, "SSI 4 Flow Setpoint"=w384:dbl)
                  n118 = Unbundle(w356) -> ("Internal Temp"=w360:dbl, "External Temp"=w359:dbl, "Power"=w361:i8, "Julabo Setpoint"=w357:dbl)
                  n119 = To Double Precision Float(number=w361) -> (double precision float=w358:dbl)
                  n120 = Cluster To Array(cluster=w362) -> (array=w382:dbl[])
                  n121 = Cluster To Array(cluster=w363) -> (array=w380:dbl[])
                  n122 = Cluster To Array(cluster=w364) -> (array=w378:dbl[])
                  n123 = Cluster To Array(cluster=w365) -> (array=w374:dbl[])
                  n124 = Cluster To Array(cluster=w366) -> (array=w372:dbl[])
                  n125 = Get Date/Time In Seconds() -> (seconds since 1Jan1904=w390:timestamp)
                  n126 = Build Array(w360, w359, w358, w357) -> (w355:dbl[])
                  n127 = Number To Fractional String(number=w382) -> (F-format string=w381:string[])  [unwired: 3 in]
                  n128 = Number To Fractional String(number=w380) -> (F-format string=w379:string[])  [unwired: 3 in]
                  n129 = Number To Fractional String(number=w378) -> (F-format string=w377:string[])  [unwired: 3 in]
                  n130 = Number To Fractional String(number=w374) -> (F-format string=w373:string[])  [unwired: 3 in]
                  n131 = Number To Fractional String(number=w372) -> (F-format string=w371:string[])  [unwired: 3 in]
                  n132 = Number To Fractional String(number=w367) -> (F-format string=w370:string[])  [unwired: 3 in]
                  n133 = Get Date/Time String(seconds (now)=w390, want seconds? (F)=TRUE) -> (date string=w392:string, time string=w393:string)  [unwired: 1 in]
                  n134 = call <vilib>:"Space Constant.vi"() -> ("String"=w394:string)
                  n135 = Build Array(w387, w386, w385, w384) -> (w376:dbl[])
                  n136 = Number To Fractional String(number=w376) -> (F-format string=w375:string[])  [unwired: 3 in]
                  n137 = Number To Fractional String(number=w355) -> (F-format string=w354:string[])  [unwired: 3 in]
                  n138 = Concatenate Strings(w392, w394, w393) -> (w383:string)
                  n139 = Build Array (concatenate)(w383, w381, w379, w377, w375, w373, w371, w370, w354) -> (w369:string[])
                  n140 = call-poly <vilib>:"Write To Spreadsheet File.vi"("delimiter (\\t)"="," ("delimiter (\\t)"), "append to file? (new file:F)"=TRUE ("append to file?"), "1D data"=w369) -> ()  [unwired: 5 in, 1 out]
                }
              }
            }
          }
        }
      }
    }
    frame #4 {
      n141 = Unbundle(w407) -> ("appended path"=w406:path)  [unwired: 4 out]
      n142 = Index Array(array=w411, index=3) -> (element=w410:cluster{i32[], i32[]})
      n143 = Unbundle(w410) -> (w412:i32[])  [unwired: 1 out]
      n144 = case shown="False" w395 {
        tunnel: w416 -> [_ w434]
        tunnel: w415 -> [_ w433]
        tunnel: w414 -> [_ w432]
        tunnel: w413 -> [_ w431]
        tunnel: w412 -> [_ w430]
        tunnel: [w417 w429] -> w408
        tunnel: w406 -> [w417 w428]
        tunnel: w405 -> [_ w427]
        tunnel: w404 -> [_ w426]
        tunnel: w403 -> [_ w425]
        tunnel: w402 -> [_ w424]
        tunnel: w401 -> [_ w423]
        tunnel: w400 -> [_ w422]
        tunnel: w399 -> [_ w421]
        tunnel: w398 -> [_ w420]
        tunnel: w397 -> [_ w419]
        tunnel: w396 -> [_ w418]
        frame False {
        }
        frame True {
          n145 = case shown="True" w431 {
            tunnel: w434 -> [_ w458]
            tunnel: w433 -> [_ w457]
            tunnel: w432 -> [_ w456]
            tunnel: w428 -> [_ w450]
            tunnel: [w443 w450] -> w429
            tunnel: w430 -> [_ w452]
            tunnel: w427 -> [w442 _]
            tunnel: w426 -> [w438 _]
            tunnel: w425 -> [_ w451]
            tunnel: w424 -> [_ w449]
            tunnel: w423 -> [_ w448]
            tunnel: w422 -> [_ w447]
            tunnel: w421 -> [_ w446]
            tunnel: w420 -> [w437 _]
            tunnel: w419 -> [_ w445]
            tunnel: w418 -> [_ w444]
            frame False {
              n146 = Build Path(base path=w442, name or relative path="Data_Product.csv" ("default name")) -> (appended path=w443:path)
              "Data_Product path" <- w443
              n147 = Number To Fractional String(number=w438) -> (F-format string=w436:string[])  [unwired: 3 in]
              n148 = Build Array (concatenate)(w437, w436) -> (w435:string[])
              n149 = call-poly <vilib>:"Write To Spreadsheet File.vi"("delimiter (\\t)"="," ("delimiter (\\t)"), "append to file? (new file:F)"=TRUE ("append to file?"), "1D data"=w435, "file path (dialog if empty)"=w443) -> ()  [unwired: 4 in, 1 out]
            }
            frame True {
              n150 = Add Array Elements(numeric array=w452) -> (sum=w455:i32)
              n151 = Not Equal?(x=w455, y=0) -> (x != y?=w453:bool)
              n152 = case shown="True" w453 {
                tunnel: w458 -> [_ _]
                tunnel: w457 -> [_ w461]
                tunnel: w456 -> [_ w462]
                tunnel: w450 -> [_ w469]
                tunnel: w452 -> [_ w468]
                tunnel: w451 -> [_ w467]
                tunnel: w449 -> [_ w466]
                tunnel: w448 -> [_ w465]
                tunnel: w447 -> [_ w463]
                tunnel: w446 -> [_ w464]
                tunnel: w445 -> [_ w460]
                tunnel: w444 -> [_ w459]
                frame False {
                }
                frame True {
                  n153 = case shown="False" w459 {
                    tunnel: w469 -> [_ w533]
                    tunnel: w468 -> [w474 w532]
                    tunnel: w467 -> [_ w524]
                    tunnel: w466 -> [w470 w518]
                    tunnel: w465 -> [w475 w515]
                    tunnel: w464 -> [w477 w514]
                    tunnel: w463 -> [w476 w511]
                    tunnel: w462 -> [w473 _]
                    tunnel: w461 -> [w472 _]
                    tunnel: w460 -> [w471 _]
                    frame False {
                      n154 = Unbundle By Name(w470) -> ("SSI 1 Flow Setpoint"=w503:dbl, "SSI 2 Flow Setpoint"=w502:dbl, "SSI 3 Flow Setpoint"=w501:dbl, "SSI 4 Flow Setpoint"=w500:dbl)
                      n155 = Unbundle(w471) -> ("Internal Temp"=w483:dbl, "External Temp"=w482:dbl, "Power"=w484:i8, "Julabo Setpoint"=w480:dbl)
                      n156 = To Double Precision Float(number=w484) -> (double precision float=w481:dbl)
                      n157 = Cluster To Array(cluster=w476) -> (array=w498:dbl[])
                      n158 = Cluster To Array(cluster=w475) -> (array=w496:dbl[])
                      n159 = Cluster To Array(cluster=w472) -> (array=w494:dbl[])
                      n160 = Cluster To Array(cluster=w473) -> (array=w490:dbl[])
                      n161 = Cluster To Array(cluster=w477) -> (array=w488:dbl[])
                      n162 = Get Date/Time In Seconds() -> (seconds since 1Jan1904=w506:timestamp)
                      n163 = Build Array(w483, w482, w481, w480) -> (w479:dbl[])
                      n164 = Number To Fractional String(number=w498) -> (F-format string=w497:string[])  [unwired: 3 in]
                      n165 = Number To Fractional String(number=w496) -> (F-format string=w495:string[])  [unwired: 3 in]
                      n166 = Number To Fractional String(number=w494) -> (F-format string=w493:string[])  [unwired: 3 in]
                      n167 = Number To Fractional String(number=w490) -> (F-format string=w489:string[])  [unwired: 3 in]
                      n168 = Number To Fractional String(number=w488) -> (F-format string=w487:string[])  [unwired: 3 in]
                      n169 = Number To Fractional String(number=w474) -> (F-format string=w486:string[])  [unwired: 3 in]
                      n170 = Get Date/Time String(seconds (now)=w506, want seconds? (F)=TRUE) -> (date string=w508:string, time string=w509:string)  [unwired: 1 in]
                      n171 = call <vilib>:"Space Constant.vi"() -> ("String"=w510:string)
                      n172 = Build Array(w503, w502, w501, w500) -> (w492:dbl[])
                      n173 = Number To Fractional String(number=w492) -> (F-format string=w491:string[])  [unwired: 3 in]
                      n174 = Number To Fractional String(number=w479) -> (F-format string=w478:string[])  [unwired: 3 in]
                      n175 = Concatenate Strings(w508, w510, w509) -> (w499:string)
                      n176 = Build Array (concatenate)(w499, w497, w495, w493, w491, w489, w487, w486, w478) -> (w485:string[])
                      n177 = call-poly <vilib>:"Write To Spreadsheet File.vi"("delimiter (\\t)"="," ("delimiter (\\t)"), "append to file? (new file:F)"=TRUE ("append to file?"), "1D data"=w485) -> ()  [unwired: 5 in, 1 out]
                    }
                    frame True {
                      w523 = 30.0  # time delay (s)
                      # "this section needs to be \nfixed to properly write data:\nit can also be done away with\nin favor of handling spectral\ndata differently if desired, \nthough it may still be worthwhile\nto output spectral data with\nsensor data"
                      # "Works for now, edit later\nto choose which data\nneeded to read in"
                      n178 = Cluster To Array(cluster=w511) -> ()  [unwired: 1 out]
                      n179 = Cluster To Array(cluster=w515) -> ()  [unwired: 1 out]
                      n180 = Cluster To Array(cluster=w514) -> ()  [unwired: 1 out]
                      n181 = Get Date/Time In Seconds() -> (seconds since 1Jan1904=w536:timestamp)
                      n182 = call <vilib>:"Space Constant.vi"() -> ("String"=w530:string)
                      n183 = Number To Fractional String(number=w532) -> (F-format string=w513:string[])  [unwired: 3 in]
                      n184 = Get Date/Time String(seconds (now)=w536, want seconds? (F)=TRUE) -> (date string=w538:string, time string=w539:string)  [unwired: 1 in]
                      n185 = Unbundle By Name(w518) -> ("SSI 1 Flow Setpoint"=w521:dbl, "SSI 2 Flow Setpoint"=w517:dbl, "SSI 3 Flow Setpoint"=w520:dbl, "SSI 4 Flow Setpoint"=w519:dbl)
                      n186 = call <vilib>:"Space Constant.vi"() -> ("String"=w540:string)
                      n187 = Concatenate Strings(w538, w540, w539) -> (w531:string)
                      n188 = call "Read_From_CSV_CFR_CWB.vi"("time delay (s)"=w523, "input string"=w531, "Spreadsheet path (.csv)"=w524) -> ("output data"=w525:string[], "time stamp"=w527:timestamp)  [unwired: 6 in]
                      n189 = Get Date/Time String(seconds (now)=w527, want seconds? (F)=TRUE) -> (date string=w522:string, time string=w529:string)  [unwired: 1 in]
                      n190 = Concatenate Strings(w522, w530, w529) -> (w526:string)
                      n191 = Build Array(w521, w517, w520, w519) -> (w516:dbl[])
                      n192 = Number To Fractional String(number=w516) -> (F-format string=w512:string[])  [unwired: 3 in]
                      n193 = Build Array (concatenate)(w526, w525, w513, w512) -> (w541:string[])
                      n194 = call-poly <vilib>:"Write To Spreadsheet File.vi"("delimiter (\\t)"="," ("delimiter (\\t)"), "append to file? (new file:F)"=TRUE ("append to file?"), "1D data"=w541, "file path (dialog if empty)"=w533) -> ()  [unwired: 4 in, 1 out]
                    }
                  }
                }
              }
            }
          }
        }
      }
    }
  }
  n195 = Bundle(cluster=w17, "appended path"=w15, "appended path"=w14, "appended path"=w13, "appended path"=w11, "appended path"=w12) -> (→"Filepath Cluster Out":T4)
